vi "MdfCreateChannel.vi"(8 "error in (no error)":errorcluster, 9 "RecordDataType":enum16{"Time", "String", "Double", "Float"}(ring), 10 "ChannelInfo":T1, 11 "ChannelGroupRef in":refnum<k24>) -> (0 "error out":errorcluster, 2 "ChannelRef":refnum<k24>, 3 "ChannelGroupRef out":refnum<k24>)   [LabVIEW 2025, in "MdfFile.lvlib"]
uses:
  MdfFile.lvlib
  data/mdflibrary.dll
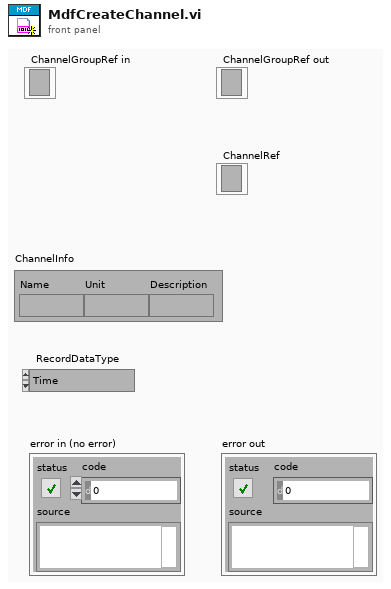
[diagram p1: front panel]
types:
  T1 = cluster{"Name":string, "Unit":string, "Description":string}
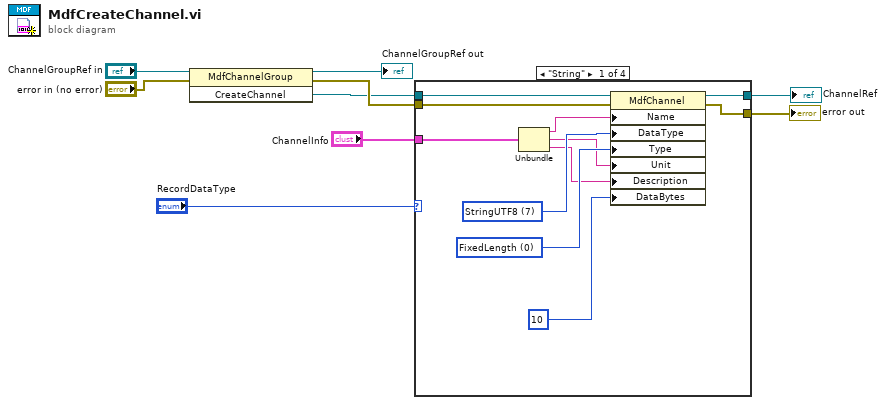
[diagram p0: block diagram]
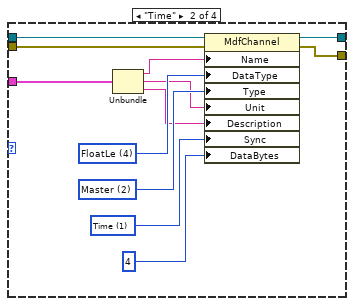
[diagram p2: hidden frame]
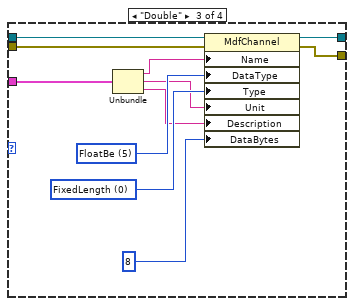
[diagram p3: hidden frame]
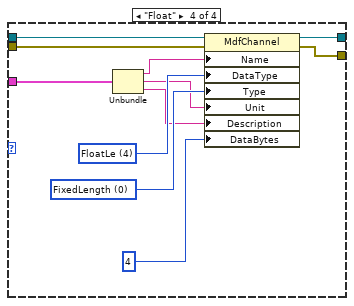
[diagram p4: hidden frame]
diagram:
  n1 = invoke class="MdfChannelGroup" method="CreateChannel"(reference="ChannelGroupRef in", error in="error in (no error)") -> (reference out=→"ChannelGroupRef out":refnum<k24>, error out=w7:errorcluster, "CreateChannel"=w4:refnum<k24>)  [unwired: 1 in]
  n2 = case shown="\"String\"" "RecordDataType" {
    tunnel: w7 -> [w20 w32 w43 w54]
    tunnel: [w19 w31 w42 w53] -> w6
    tunnel: [w18 w30 w41 w52] -> w5
    tunnel: w4 -> [w17 w29 w40 w51]
    tunnel: "ChannelInfo" -> [w10 w21 w33 w44]
    frame "String" {
      w15 = u8 0 items=["FixedLength", "VariableLength", "Master", "VirtualMaster", "Sync", "MaxLength", "VirtualData"] ("Type")
      w16 = u8 7 items=["UnsignedIntegerLe", "UnsignedIntegerBe", "SignedIntegerLe", "SignedIntegerBe", "FloatLe", "FloatBe", "StringAscii", "StringUTF8", "StringUTF16Le", "StringUTF16Be", "ByteArray", "MimeSample", "MimeStream", "CanOpenDate", "CanOpenTime", "ComplexLe", "ComplexBE"] ("DataType")
      n3 = Unbundle(w10) -> ("Name"=w14:string, "Unit"=w13:string, "Description"=w12:string)
      n4 = property class="MdfChannel"(reference=w17, error in=w20, "Name"=w14, "DataType"=w16, "Type"=w15, "Unit"=w13, "Description"=w12, "DataBytes"=u64 10) -> (reference out=w18:refnum<k24>, error out=w19:errorcluster)
    }
    frame "Time" {
      w23 = u8 1 items=["None", "Time", "Angle", "Distance", "Index"] ("Sync")
      w27 = u8 2 items=["FixedLength", "VariableLength", "Master", "VirtualMaster", "Sync", "MaxLength", "VirtualData"] ("Type")
      w28 = u8 4 items=["UnsignedIntegerLe", "UnsignedIntegerBe", "SignedIntegerLe", "SignedIntegerBe", "FloatLe", "FloatBe", "StringAscii", "StringUTF8", "StringUTF16Le", "StringUTF16Be", "ByteArray", "MimeSample", "MimeStream", "CanOpenDate", "CanOpenTime", "ComplexLe", "ComplexBE"] ("DataType")
      n5 = Unbundle(w21) -> ("Name"=w26:string, "Unit"=w25:string, "Description"=w24:string)
      n6 = property class="MdfChannel"(reference=w29, error in=w32, "Name"=w26, "DataType"=w28, "Type"=w27, "Unit"=w25, "Description"=w24, "Sync"=w23, "DataBytes"=u64 4) -> (reference out=w30:refnum<k24>, error out=w31:errorcluster)
    }
    frame "Double" {
      w38 = u8 0 items=["FixedLength", "VariableLength", "Master", "VirtualMaster", "Sync", "MaxLength", "VirtualData"] ("Type")
      w39 = u8 5 items=["UnsignedIntegerLe", "UnsignedIntegerBe", "SignedIntegerLe", "SignedIntegerBe", "FloatLe", "FloatBe", "StringAscii", "StringUTF8", "StringUTF16Le", "StringUTF16Be", "ByteArray", "MimeSample", "MimeStream", "CanOpenDate", "CanOpenTime", "ComplexLe", "ComplexBE"] ("DataType")
      n7 = Unbundle(w33) -> ("Name"=w37:string, "Unit"=w36:string, "Description"=w35:string)
      n8 = property class="MdfChannel"(reference=w40, error in=w43, "Name"=w37, "DataType"=w39, "Type"=w38, "Unit"=w36, "Description"=w35, "DataBytes"=u64 8) -> (reference out=w41:refnum<k24>, error out=w42:errorcluster)
    }
    frame "Float" {
      w49 = u8 0 items=["FixedLength", "VariableLength", "Master", "VirtualMaster", "Sync", "MaxLength", "VirtualData"] ("Type")
      w50 = u8 4 items=["UnsignedIntegerLe", "UnsignedIntegerBe", "SignedIntegerLe", "SignedIntegerBe", "FloatLe", "FloatBe", "StringAscii", "StringUTF8", "StringUTF16Le", "StringUTF16Be", "ByteArray", "MimeSample", "MimeStream", "CanOpenDate", "CanOpenTime", "ComplexLe", "ComplexBE"] ("DataType")
      n9 = Unbundle(w44) -> ("Name"=w48:string, "Unit"=w47:string, "Description"=w46:string)
      n10 = property class="MdfChannel"(reference=w51, error in=w54, "Name"=w48, "DataType"=w50, "Type"=w49, "Unit"=w47, "Description"=w46, "DataBytes"=u64 4) -> (reference out=w52:refnum<k24>, error out=w53:errorcluster)
    }
  }
  "error out" <- w6
  "ChannelRef" <- w5
